vi "SampleDataDlg.vi"(9 "采样数据in":string[][](array[string]), 10 "采样区域in":string, 11 "采样时间in":string) -> (3 "采样数据":string[][](array[string]))   [LabVIEW 2014, in "Sample.lvlib"]
uses:
  Sample/Sample.lvlib
panel:
  out "保存数据路径":path
  in  "导出数据":bool
  out "采样区域":string
  out "采样时间":string
  in  "采样数据":i32(listbox)
  in  "退出":bool
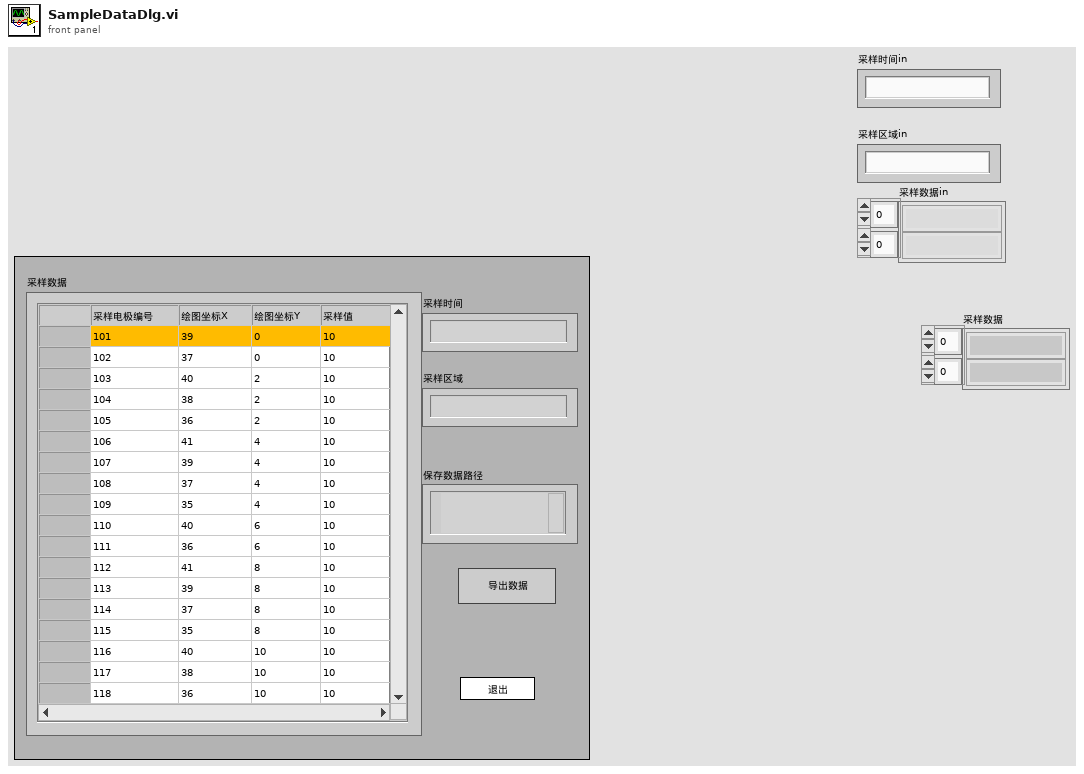
[diagram p1: front panel]
types:
  T1 = enum32{"invalid app kind", "Development System", "Run Time System", "Student Edition", "Embedded LabVIEW", "Evaluation", "Custom"}
  T2 = enum32{"Invalid", "Standard", "Closed", "Hidden", "Minimized", "Maximized"}
  T3 = cluster{"Core":cluster{"Current VI Reference":refnum<vi>, "Close Panel on Exit?":bool}, "Your Boolean data":bool, "Your string data":string, "采样数据":string[][], "采样区域":string, "采样时间":string}
  T4 = cluster{"Current VI Reference":refnum<vi>, "Close Panel on Exit?":bool}
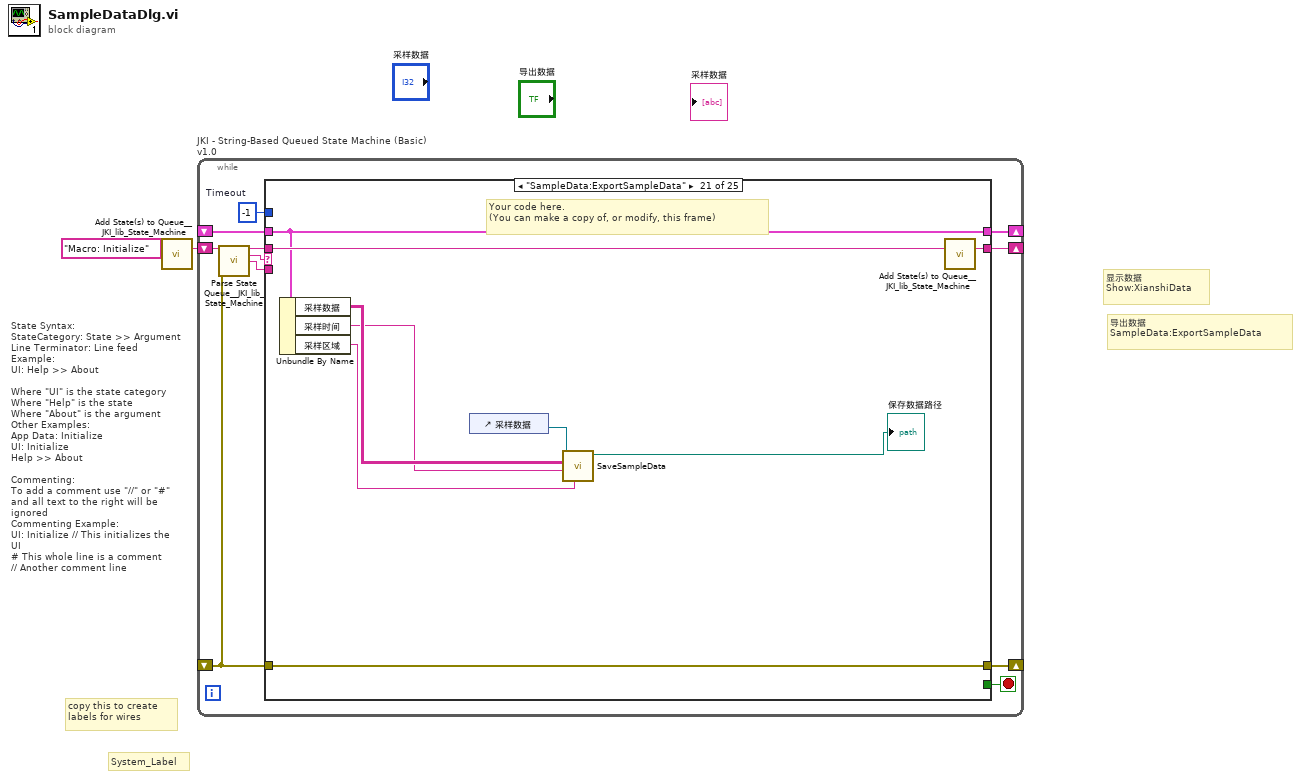
[diagram p0: block diagram]
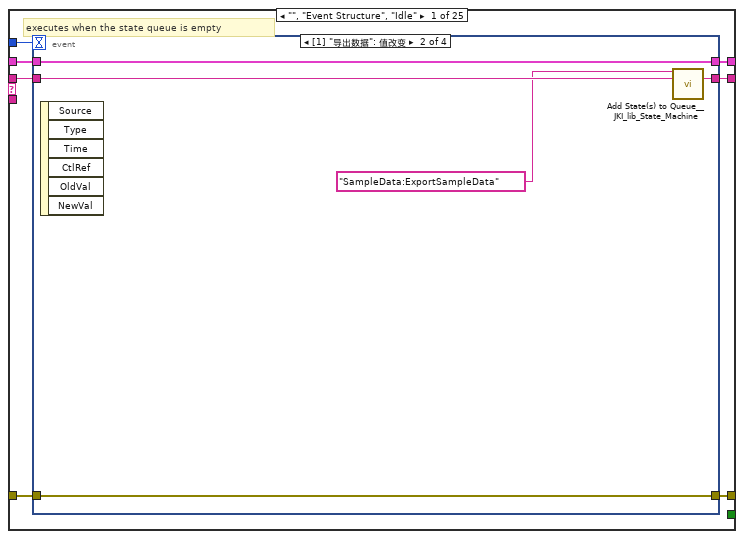
[diagram p2: hidden frame]
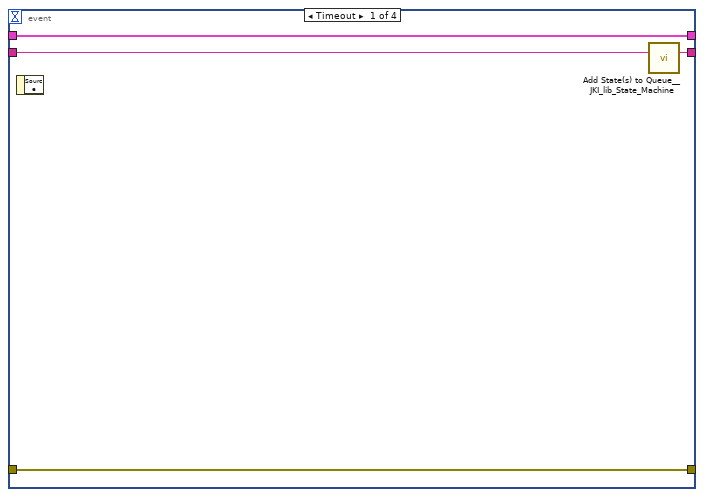
[diagram p3: hidden frame]
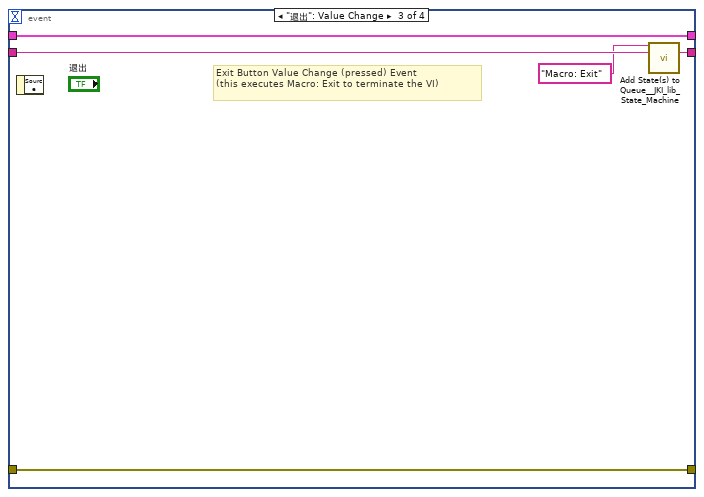
[diagram p4: hidden frame]
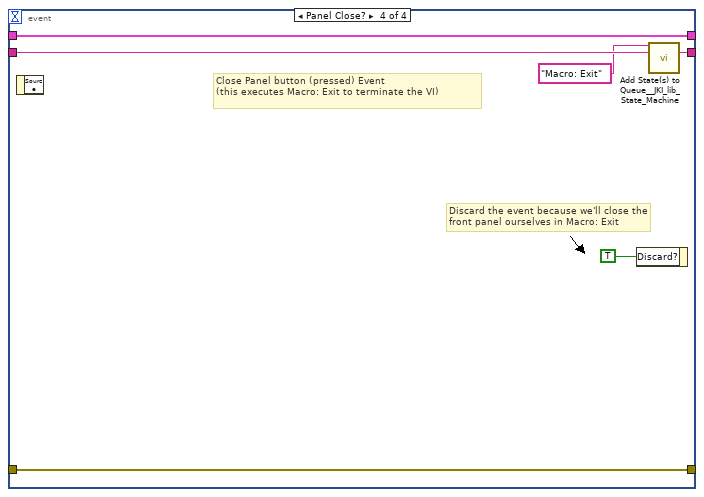
[diagram p5: hidden frame]
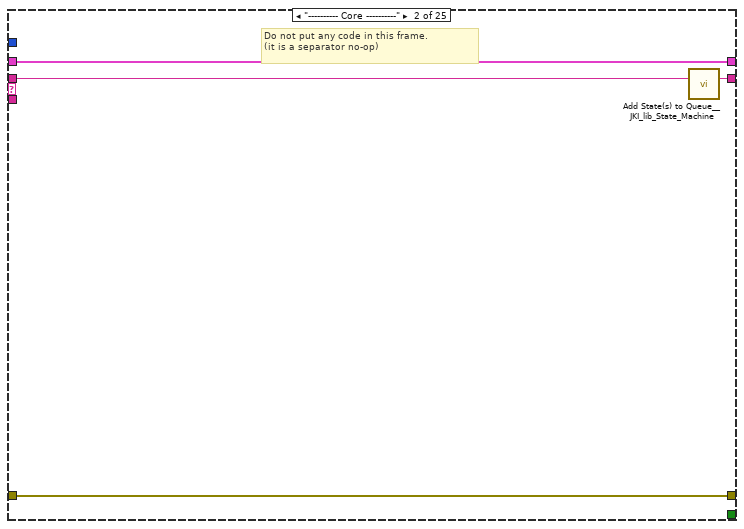
[diagram p6: hidden frame]
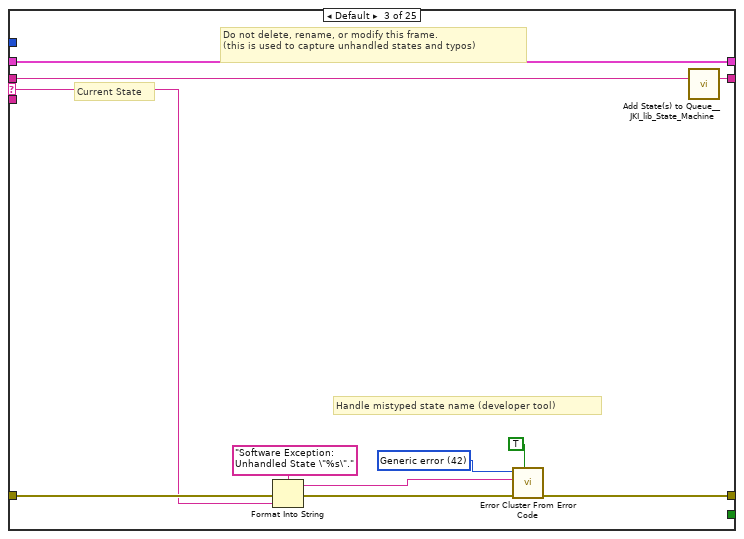
[diagram p7: hidden frame]
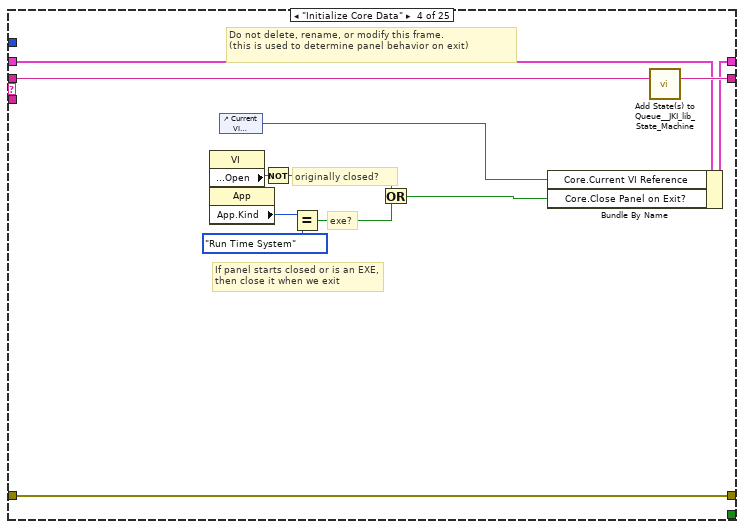
[diagram p8: hidden frame]
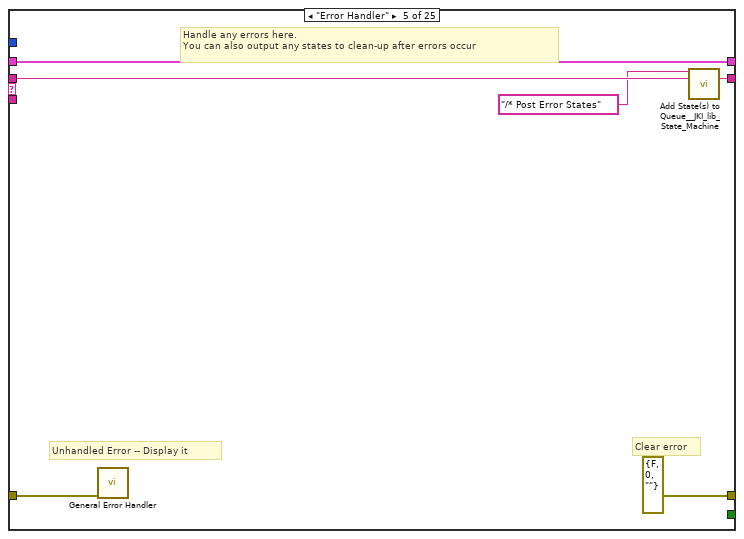
[diagram p9: hidden frame]
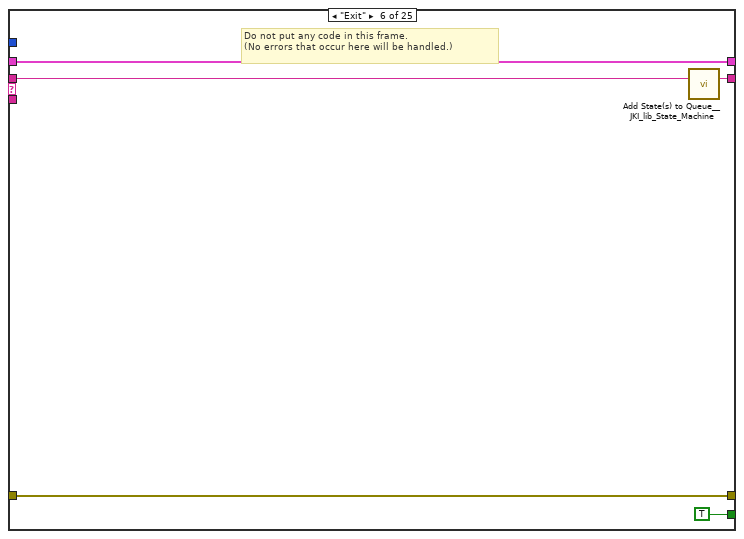
[diagram p10: hidden frame]
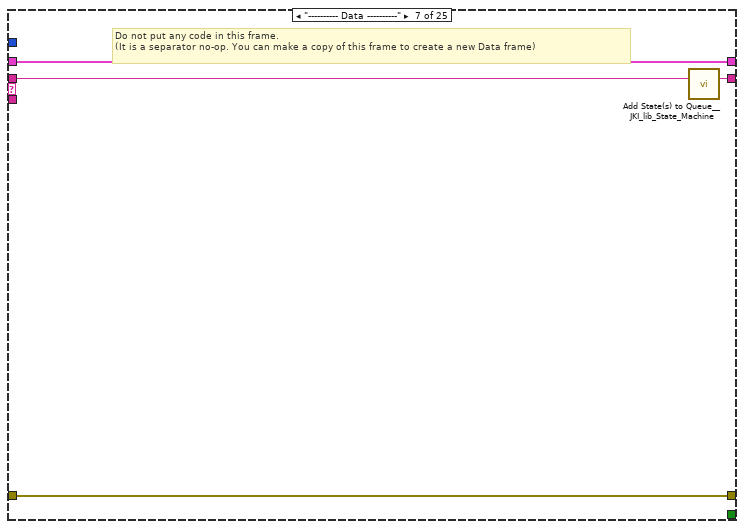
[diagram p11: hidden frame]
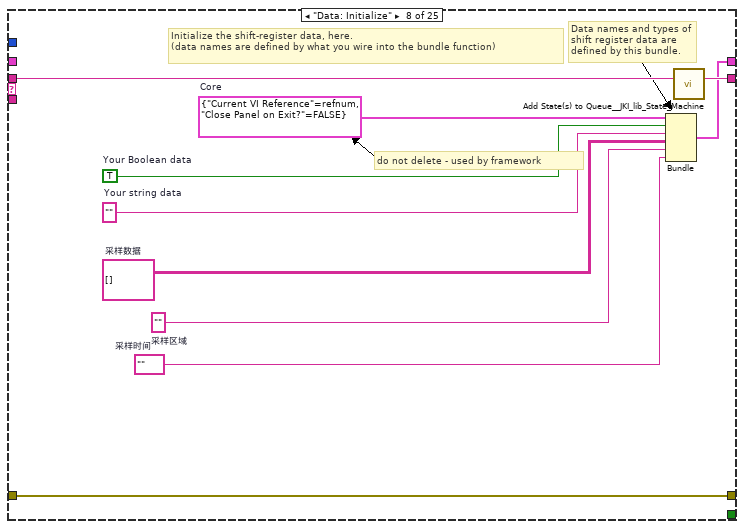
[diagram p12: hidden frame]
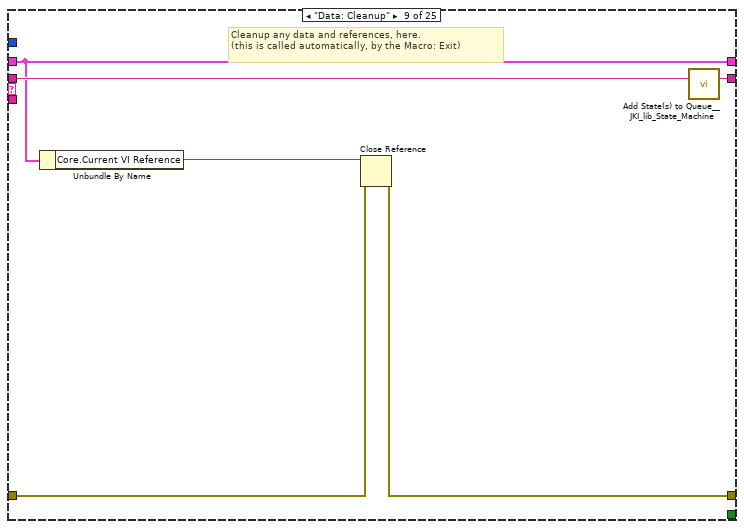
[diagram p13: hidden frame]
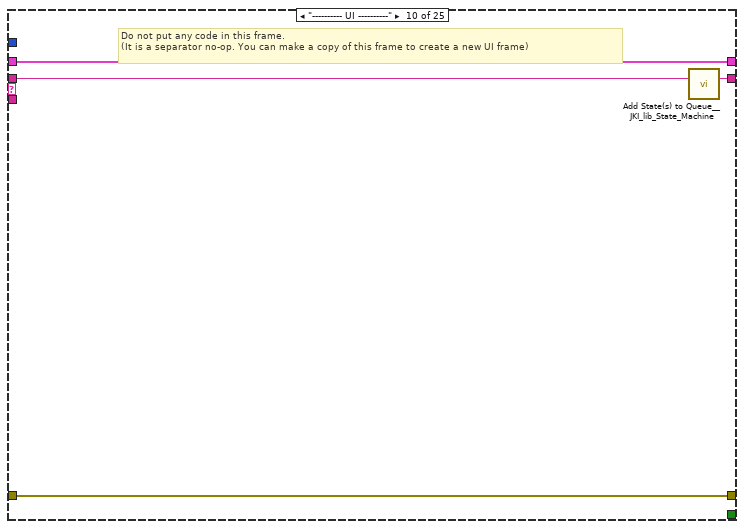
[diagram p14: hidden frame]
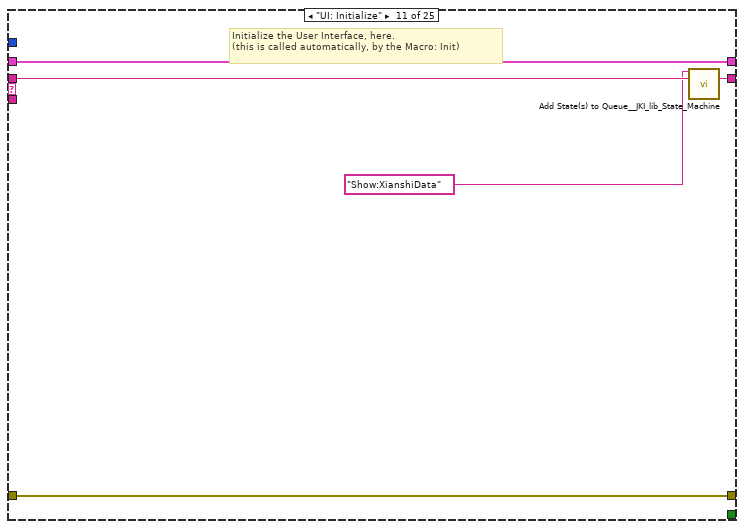
[diagram p15: hidden frame]
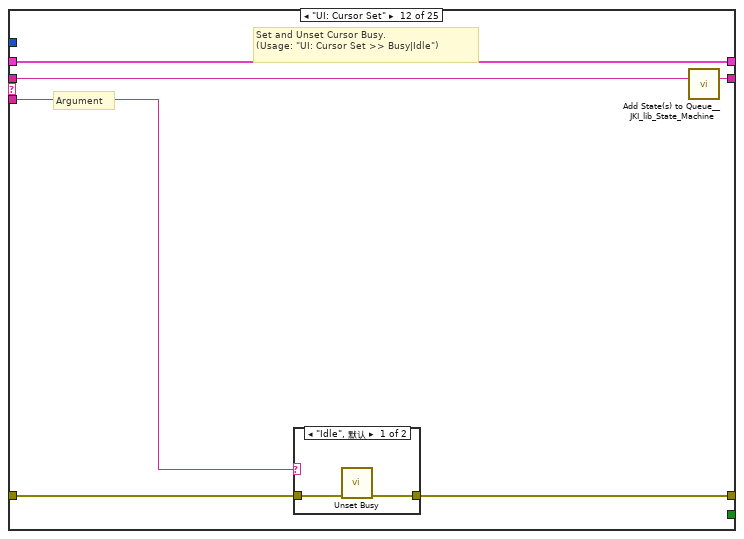
[diagram p16: hidden frame]
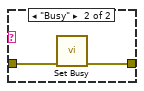
[diagram p17: hidden frame]
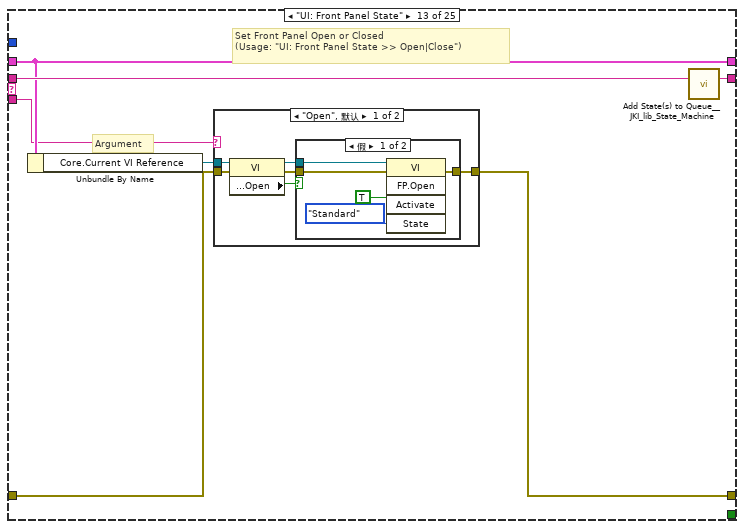
[diagram p18: hidden frame]
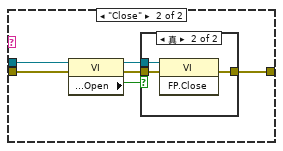
[diagram p20: hidden frame]
diagram:
  # "导出数据\nSampleData:ExportSampleData"
  # "显示数据\nShow:XianshiData"
  # "State Syntax:\nStateCategory: State >> Argument\nLine Terminator: Line feed\nExample:\nUI: Help >> About\n\nWhere \"UI\" is the state category\nWhere \"Help\" is the state\nWhere \"About\" is the argument\nOther Examples:\nApp Data: Initialize\nUI: Initialize\nHelp >> About\n\nCommenting:\nTo add a comment use \"//\" or \"#\" and all text to the right will be ignored\nCommenting Example:\nUI: Initialize // This initializes the UI\n# This whole line is a comment\n// Another comment line"
  # "copy this to create labels for wires"
  # "System_Label"
  n1 = call <vilib>:"Add State(s) to Queue__JKI_lib_State_Machine.vi"("State(s) in (\"\")"="Macro: Initialize") -> ("States Out"=w2:string)  [unwired: 14 in]
  n2 = while "JKI - String-Based Queued State Machine (Basic) v1.0" {
    shift-right: [w6] -> _
    shift-left: _ -> [w5]
    shift-right: [w9] -> _
    shift-left: _ -> [w3]
    shift-right: [w8] -> _
    shift-left: w2 -> [w10]
    stop <- w7 stop-if-true
    w4 = -1  # Timeout
    n3 = call <vilib>:"Parse State Queue__JKI_lib_State_Machine.vi"("State Queue"=w10, "Error In (no error)"=w3) -> ("Remaining States"=w12:string, "Current State"=w13:string, "Arguments"=w11:string)  [unwired: 11 in]
    n4 = case shown="\"SampleData:ExportSampleData\"" w13 {
      selector: w13 -> [_ _ w45 _ _ _ _ _ _ _ _ _ _ _ _ _ _ _ _ _ _ _ _ _ _]
      tunnel: w12 -> [w20 w44 w49 w67 w73 w78 w82 w92 w98 w102 w107 w113 w124 w150 w155 w165 w169 w173 w177 w181 w190 w194 w201 w205 w213]
      tunnel: w11 -> [_ _ _ _ _ _ _ _ _ _ _ w108 w118 _ _ _ _ _ _ _ _ _ _ _ _]
      tunnel: w5 -> [w18 w41 w47 w58 w70 w76 w79 _ w93 w99 w105 w111 w120 w147 w152 w162 w166 w170 w174 w178 w187 w191 w198 w202 w210]
      tunnel: [w17 w42 w51 w64 errorcluster {"status"=FALSE, "code"=0, "source"=""} ("error out") w75 w80 w89 w94 w100 w104 w109 w121 w148 w153 w163 w167 w171 w175 w179 w188 w192 w199 w203 w211] -> w9
      tunnel: w3 -> [w16 w42 w50 w64 w69 w75 w80 w89 w95 w100 w104 w110 w122 w148 w153 w163 w167 w171 w175 w179 w188 w192 w199 w203 w211]
      tunnel: [w19 w43 w48 w66 w72 w77 w81 w91 w97 w101 w106 w112 w123 w149 w154 w164 w168 w172 w176 w180 w189 w193 w200 w204 w212] -> w8
      tunnel: [_ _ _ _ _ TRUE _ _ _ _ _ _ _ _ _ _ _ _ _ _ _ _ _ _ _] -> w7
      tunnel: [w15 w41 w47 w65 w70 w76 w79 w90 w93 w99 w105 w111 w120 w147 w152 w162 w166 w170 w174 w178 w187 w191 w198 w202 w209] -> w6
      tunnel: w4 -> [w14 _ _ _ _ _ _ _ _ _ _ _ _ _ _ _ _ _ _ _ _ _ _ _ _]
      frame "", "Event Structure", "Idle" {
        # "executes when the state queue is empty"
        n5 = event shown="[1] \"导出数据\": 值改变" {
          selector: _ -> [_ _ _ _]
          dyn-events: _ -> [_ _ _ _]
          timeout: w14 -> [_ _ _ _]
          tunnel: w20 -> [w24 w29 w34 w40]
          tunnel: [w23 w28 w33 w39] -> w19
          tunnel: w18 -> [w21 w26 w31 w37]
          tunnel: [w22 w27 w32 w38] -> w17
          tunnel: w16 -> [w22 w27 w32 w38]
          tunnel: [w21 w26 w31 w37] -> w15
          event Timeout {
            n6 = event-data() -> ()  [unwired: 1 in, 1 out]
            n7 = call <vilib>:"Add State(s) to Queue__JKI_lib_State_Machine.vi"("State(s) in (\"\")"=w24) -> ("States Out"=w23:string)  [unwired: 14 in]
          }
          event "导出数据": Value Change {
            n8 = event-data() -> ()  [unwired: 1 in, 6 out]
            n9 = call <vilib>:"Add State(s) to Queue__JKI_lib_State_Machine.vi"("State(s) in Front (\"\")"="SampleData:ExportSampleData", "State(s) in (\"\")"=w29) -> ("States Out"=w28:string)  [unwired: 13 in]
          }
          event "退出": Value Change {
            # "Exit Button Value Change (pressed) Event\n(this executes Macro: Exit to terminate the VI)"
            n10 = event-data() -> ()  [unwired: 1 in, 1 out]
            n11 = call <vilib>:"Add State(s) to Queue__JKI_lib_State_Machine.vi"("State(s) in Front (\"\")"="Macro: Exit", "State(s) in (\"\")"=w34) -> ("States Out"=w33:string)  [unwired: 13 in]
          }
          event Panel Close? {
            # "Discard the event because we'll close the front panel ourselves in Macro: Exit"
            # "Close Panel button (pressed) Event\n(this executes Macro: Exit to terminate the VI)"
            n12 = event-data() -> ()  [unwired: 1 in, 1 out]
            n13 = event-data("Discard?"=TRUE) -> ()  [unwired: 1 in, 1 out]
            n14 = call <vilib>:"Add State(s) to Queue__JKI_lib_State_Machine.vi"("State(s) in Front (\"\")"="Macro: Exit", "State(s) in (\"\")"=w40) -> ("States Out"=w39:string)  [unwired: 13 in]
          }
        }
      }
      frame "---------- Core ----------" {
        # "Do not put any code in this frame.\n(it is a separator no-op)"
        n15 = call <vilib>:"Add State(s) to Queue__JKI_lib_State_Machine.vi"("State(s) in (\"\")"=w44) -> ("States Out"=w43:string)  [unwired: 14 in]
      }
      frame Default {
        w54 = 42 items=["No error", "Argument error", "Memory is full", "Out of zone", "End of file", "File already open", "Generic file I/O error", "File not found", "File permission error", "Disk is full", "Duplicate path", "Too many files open", "System feature not enabled", "Resource file not found", "Cannot add resource", "Resource not found", "Image not found", "Image memory error", "Pen does not exist", "Config type invalid", "Config token not found", "Config parse error", "Config memory error", "Bad external code format", "Bad external code offset", "External code not present", "Null window", "Destroy window error", "Null menu", "Print aborted", "Bad print record", "Print driver error", "Windows error during printing", "Memory error during printing", "Print dialog error", "Generic print error", "Invalid device refnum", "Device not found", "Device parameter error", "Device unit error", "Cannot open device", "Device call aborted", "Generic error", "Cancelled by user", "Object ID too low", "Object ID too high", "Object not in heap", "Unknown heap", "Unknown object (invalid DefProc)", "Unknown object (DefProc not in table)", "Message out of range", "Invalid (null) method", "Unknown message", "Manager call not supported", "Bad address", "Network operation in progress", "Network operation timed out", "Connection is busy", "Network attribute not supported", "Network error", "Address in use", "System out of memory", "Connection aborted", "Connection refused", "Not connected", "Already connected", "Connection closed", "Initialization error (interapplication manager)", "Bad occurrence", "Wait on unbound occurrence handler", "Occurrence queue overflow", "Datalog type conflict", "Unused", "Unrecognized type (interapplication manager)", "Memory corrupt", "Failed to make temporary DLL", "Old CIN version", "Drag socket not found", "Failed to load drop-object", "Failed to register OLE object", "Failed to release OLE object", "Format specifier type mismatch", "Unknown format specifier", "Too few format specifiers", "Too many format specifiers", "Scan failed", "Newer CIN version", "Error converting to variant", "Runtime menu error", "Password tampered", "Variant attribute not found", "Incompatible variant data type", "Event data is not available", "Event Store is not present", "Occurrence is not found", "Event Queue is not created", "Event info is not available", "Refnum passed is NULL", "Error retrieving Class GUID", "Error retrieving CoClass GUID", "Error retrieving TypeLib GUID.", "Bad built application magic bytes.", "Specific driver is different from the specific driver associated with the Logical Name.", "There is no session opened to the class driver.", "Max Error", "MAX - Error with config objects", "MAX - Error loading configuration", "MAX - Group not supported"]
        # "Current State"
        # "Do not delete, rename, or modify this frame.\n(this is used to capture unhandled states and typos)"
        # "Handle mistyped state name (developer tool)"
        n16 = Format Into String(format string="Software Exception: Unhandled State \"%s\"." ("message"), error in=w50, w45) -> (resulting string=w53:string, error out=w52:errorcluster)  [unwired: 1 in]
        n17 = call <vilib>:"Error Cluster From Error Code.vi"("show call chain? (False)"=TRUE, "error in (no error)"=w52, "error message (\"\")"=w53, "error code (0)"=w54) -> ("error out"=w51:errorcluster)  [unwired: 5 in]
        n18 = call <vilib>:"Add State(s) to Queue__JKI_lib_State_Machine.vi"("State(s) in (\"\")"=w49) -> ("States Out"=w48:string)  [unwired: 14 in]
      }
      frame "Initialize Core Data" {
        # "Do not delete, rename, or modify this frame.\n(this is used to determine panel behavior on exit)"
        # "originally closed?"
        # "exe?"
        # "If panel starts closed or is an EXE, then close it when we exit"
        n19 = property class="VI"() -> ("Front Panel.Open"=w63:bool)  [unwired: 2 in, 2 out]
        n20 = property class="App"() -> ("App.Kind"=w62:T1)  [unwired: 2 in, 2 out]
        n21 = control-ref of="Current VI Reference"() -> (w56:refnum<vi>)
        n22 = Not(x=w63) -> (.not. x?=w60:bool)
        n23 = Equal?(x=w62, y=T1."Run Time System" ("Application:Kind")) -> (x = y?=w59:bool)
        n24 = Or(x=w60, y=w59) -> (x .or. y?=w57:bool)
        n25 = Bundle By Name(cluster=w58, "Core.Current VI Reference"=w56, "Core.Close Panel on Exit?"=w57) -> (w65:T3)
        n26 = call <vilib>:"Add State(s) to Queue__JKI_lib_State_Machine.vi"("State(s) in (\"\")"=w67) -> ("States Out"=w66:string)  [unwired: 14 in]
      }
      frame "Error Handler" {
        # "Unhandled Error -- Display it"
        # "Handle any errors here.\nYou can also output any states to clean-up after errors occur"
        # "Clear error"
        n27 = call <vilib>:"General Error Handler.vi"("error in (no error)"=w69) -> ()  [unwired: 10 in, 5 out]
        n28 = call <vilib>:"Add State(s) to Queue__JKI_lib_State_Machine.vi"("State(s) in Front (\"\")"="/* Post Error States", "State(s) in (\"\")"=w73) -> ("States Out"=w72:string)  [unwired: 13 in]
      }
      frame "Exit" {
        # "Do not put any code in this frame.\n(No errors that occur here will be handled.)"
        n29 = call <vilib>:"Add State(s) to Queue__JKI_lib_State_Machine.vi"("State(s) in (\"\")"=w78) -> ("States Out"=w77:string)  [unwired: 14 in]
      }
      frame "---------- Data ----------" {
        # "Do not put any code in this frame.\n(It is a separator no-op. You can make a copy of this frame to create a new Data frame)"
        n30 = call <vilib>:"Add State(s) to Queue__JKI_lib_State_Machine.vi"("State(s) in (\"\")"=w82) -> ("States Out"=w81:string)  [unwired: 14 in]
      }
      frame "Data: Initialize" {
        w83 = ""  # 采样时间
        w84 = ""  # 采样区域
        w85 = string[][] []  # 采样数据
        w86 = T4 {"Current VI Reference"=refnum, "Close Panel on Exit?"=FALSE}  # Core
        w88 = TRUE  # Your Boolean data
        w87 = ""  # Your string data
        # "do not delete - used by framework"
        # "Data names and types of shift register data are defined by this bundle."
        # "Initialize the shift-register data, here.\n(data names are defined by what you wire into the bundle function)"
        n31 = Bundle("Core"=w86, "Your Boolean data"=w88, "Your string data"=w87, "采样数据"=w85, "采样区域"=w84, "采样时间"=w83) -> (w90:T3)  [unwired: 1 in]
        n32 = call <vilib>:"Add State(s) to Queue__JKI_lib_State_Machine.vi"("State(s) in (\"\")"=w92) -> ("States Out"=w91:string)  [unwired: 14 in]
      }
      frame "Data: Cleanup" {
        # "Cleanup any data and references, here.\n(this is called automatically, by the Macro: Exit)"
        n33 = Unbundle By Name(w93) -> ("Core.Current VI Reference"=w96:refnum<vi>)
        n34 = Close Reference(reference=w96, error in (no error)=w95) -> (error out=w94:errorcluster)
        n35 = call <vilib>:"Add State(s) to Queue__JKI_lib_State_Machine.vi"("State(s) in (\"\")"=w98) -> ("States Out"=w97:string)  [unwired: 14 in]
      }
      frame "---------- UI ----------" {
        # "Do not put any code in this frame.\n(It is a separator no-op. You can make a copy of this frame to create a new UI frame)"
        n36 = call <vilib>:"Add State(s) to Queue__JKI_lib_State_Machine.vi"("State(s) in (\"\")"=w102) -> ("States Out"=w101:string)  [unwired: 14 in]
      }
      frame "UI: Initialize" {
        # "Initialize the User Interface, here.\n(this is called automatically, by the Macro: Init)"
        n37 = call <vilib>:"Add State(s) to Queue__JKI_lib_State_Machine.vi"("State(s) in Front (\"\")"="Show:XianshiData", "State(s) in (\"\")"=w107) -> ("States Out"=w106:string)  [unwired: 13 in]
      }
      frame "UI: Cursor Set" {
        # "Argument"
        # "Set and Unset Cursor Busy.\n(Usage: \"UI: Cursor Set >> Busy|Idle\")"
        n38 = case shown="\"Idle\", 默认" w108 {
          tunnel: w110 -> [w115 w117]
          tunnel: [w114 w116] -> w109
          frame "Idle", Default {
            n39 = call <vilib>:"Unset Busy.vi"("error in (no error)"=w115) -> ("error out"=w114:errorcluster)  [unwired: 10 in]
          }
          frame "Busy" {
            n40 = call <vilib>:"Set Busy.vi"("error in (no error)"=w117) -> ("error out"=w116:errorcluster)  [unwired: 9 in, 1 out]
          }
        }
        n41 = call <vilib>:"Add State(s) to Queue__JKI_lib_State_Machine.vi"("State(s) in (\"\")"=w113) -> ("States Out"=w112:string)  [unwired: 14 in]
      }
      frame "UI: Front Panel State" {
        # "Argument"
        # "Set Front Panel Open or Closed\n(Usage: \"UI: Front Panel State >> Open|Close\")"
        n42 = Unbundle By Name(w120) -> ("Core.Current VI Reference"=w119:refnum<vi>)
        n43 = case shown="\"Open\", 默认" w118 {
          tunnel: w122 -> [w128 w141]
          tunnel: [w130 w142] -> w121
          tunnel: w119 -> [w129 w139]
          frame "Open", Default {
            n44 = property class="VI"(reference=w129, error in=w128) -> (reference out=w126:refnum<vi>, error out=w127:errorcluster, "Front Panel.Open"=w125:bool)
            n45 = case shown="假" w125 {
              tunnel: [w133 w136] -> w130
              tunnel: w127 -> [w132 w136]
              tunnel: w126 -> [w131 _]
              frame False {
                n46 = invoke class="VI" method="FP.Open"(reference=w131, error in=w132, "Activate"=TRUE, "State"=T2."Standard") -> (error out=w133:errorcluster)  [unwired: 1 in, 4 out]
              }
              frame True {
              }
            }
          }
          frame "Close" {
            n47 = property class="VI"(reference=w139, error in=w141) -> (reference out=w138:refnum<vi>, error out=w140:errorcluster, "Front Panel.Open"=w137:bool)
            n48 = case shown="真" w137 {
              tunnel: [w143 w146] -> w142
              tunnel: w140 -> [w143 w145]
              tunnel: w138 -> [_ w144]
              frame False {
              }
              frame True {
                n49 = invoke class="VI" method="FP.Close"(reference=w144, error in=w145) -> (error out=w146:errorcluster)  [unwired: 1 in, 2 out]
              }
            }
          }
        }
        n50 = call <vilib>:"Add State(s) to Queue__JKI_lib_State_Machine.vi"("State(s) in (\"\")"=w124) -> ("States Out"=w123:string)  [unwired: 14 in]
      }
      frame "---------- Macro ----------" {
        # "Do not put any code in this frame.\n(It is a separator no-op. You can make a copy of this frame to create a new Macro frame)"
        n51 = call <vilib>:"Add State(s) to Queue__JKI_lib_State_Machine.vi"("State(s) in (\"\")"=w150) -> ("States Out"=w149:string)  [unwired: 14 in]
      }
      frame "Macro: Initialize" {
        w151 = "Data: Initialize\nInitialize Core Data\nSample:SampleInfo\nUI: Initialize\nUI: Front Panel State >> Open"  # Data: Initialize Initialize Core Data Sample:SampleInfo UI: Initialize UI: Front Panel State >> Open
        # "Initialization Macro\n(This is called once, when the VI starts)"
        n52 = call <vilib>:"Add State(s) to Queue__JKI_lib_State_Machine.vi"("State(s) in Front (\"\")"=w151, "State(s) in (\"\")"=w155) -> ("States Out"=w154:string)  [unwired: 13 in]
      }
      frame "Macro: Exit" {
        # "Exit Macro\n(This is called once, when the VI exits)"
        n53 = Unbundle By Name(w162) -> ("Core.Close Panel on Exit?"=w161:bool)
        n54 = Select(t="UI: Front Panel State >> Close", s=w161, f="") -> (s? t:f=w158:string)
        n55 = call <vilib>:"Add State(s) to Queue__JKI_lib_State_Machine.vi"("State(s) in (\"\")"=w158, "State(s) at Back (\"\")"="Data: Cleanup\nExit") -> ("States Out"=w156:string)  [unwired: 13 in]
        n56 = call <vilib>:"Add State(s) to Queue__JKI_lib_State_Machine.vi"("State(s) in Front (\"\")"=w156, "State(s) in (\"\")"=w165) -> ("States Out"=w164:string)  [unwired: 13 in]
      }
      frame "---------- New Category ----------" {
        # "Template Separator\n(You can make a copy of, or modify, this frame)"
        n57 = call <vilib>:"Add State(s) to Queue__JKI_lib_State_Machine.vi"("State(s) in (\"\")"=w169) -> ("States Out"=w168:string)  [unwired: 14 in]
      }
      frame "New Category: 1" {
        # "Your code here.\n(You can make a copy of, or modify, this frame)"
        n58 = call <vilib>:"Add State(s) to Queue__JKI_lib_State_Machine.vi"("State(s) in (\"\")"=w173) -> ("States Out"=w172:string)  [unwired: 14 in]
      }
      frame "New Category: 2" {
        # "Your code here.\n(You can make a copy of, or modify, this frame)"
        n59 = call <vilib>:"Add State(s) to Queue__JKI_lib_State_Machine.vi"("State(s) in (\"\")"=w177) -> ("States Out"=w176:string)  [unwired: 14 in]
      }
      frame "--------SampleData--------" {
        # "Your code here.\n(You can make a copy of, or modify, this frame)"
        n60 = call <vilib>:"Add State(s) to Queue__JKI_lib_State_Machine.vi"("State(s) in (\"\")"=w181) -> ("States Out"=w180:string)  [unwired: 14 in]
      }
      frame "SampleData:ExportSampleData" {
        # "Your code here.\n(You can make a copy of, or modify, this frame)"
        n61 = Unbundle By Name(w187) -> ("采样数据"=w186:string[][], "采样时间"=w185:string, "采样区域"=w184:string)
        n62 = control-ref of="采样数据"() -> (w183:refnum<vi>)
        n63 = call "SaveSampleData.vi"("采样区域"=w184, "采样时间"=w185, "采样数据"=w186, "MulticolumnListbox输入"=w183) -> ("保存数据路径"=→"保存数据路径":path)  [unwired: 7 in]
        n64 = call <vilib>:"Add State(s) to Queue__JKI_lib_State_Machine.vi"("State(s) in (\"\")"=w190) -> ("States Out"=w189:string)  [unwired: 14 in]
      }
      frame "-----Show------" {
        # "Your code here.\n(You can make a copy of, or modify, this frame)"
        n65 = call <vilib>:"Add State(s) to Queue__JKI_lib_State_Machine.vi"("State(s) in (\"\")"=w194) -> ("States Out"=w193:string)  [unwired: 14 in]
      }
      frame "Show:XianshiData" {
        # "Your code here.\n(You can make a copy of, or modify, this frame)"
        n66 = Unbundle By Name(w198) -> ("采样数据"=w195:string[][], "采样区域"=→"采样区域":string, "采样时间"=→"采样时间":string)
        n67 = property on="采样数据" class="MCListbox (严格)"("ItemNames"=w195) -> ()  [unwired: 2 in, 2 out]
        n68 = call <vilib>:"Add State(s) to Queue__JKI_lib_State_Machine.vi"("State(s) in (\"\")"=w201) -> ("States Out"=w200:string)  [unwired: 14 in]
      }
      frame "-------Sample-----" {
        # "Your code here.\n(You can make a copy of, or modify, this frame)"
        n69 = call <vilib>:"Add State(s) to Queue__JKI_lib_State_Machine.vi"("State(s) in (\"\")"=w205) -> ("States Out"=w204:string)  [unwired: 14 in]
      }
      frame "Sample:SampleInfo" {
        # "Your code here.\n只运行一次"
        n70 = Bundle By Name(cluster=w210, "采样数据"="采样数据in", "采样区域"="采样区域in", "采样时间"="采样时间in") -> (w209:T3)
        n71 = call <vilib>:"Add State(s) to Queue__JKI_lib_State_Machine.vi"("State(s) in (\"\")"=w213) -> ("States Out"=w212:string)  [unwired: 14 in]
      }
    }
  }
